vi "Mavlink Message Read.vi"(8 "error_in":errorcluster, 11 "VISA in":refnum<visa-resource-name>) -> (0 "error_out":errorcluster, 2 "mav_msg":T2, 3 "VISA out":refnum<visa-resource-name>)   [LabVIEW 2023]
panel:
  out "crc_counter":u32
  out "packet_counter":u32
  out "mav_msg_array":T1(array[cluster])
  out "check_mav_msg_array":bool
  out "CRC":bool
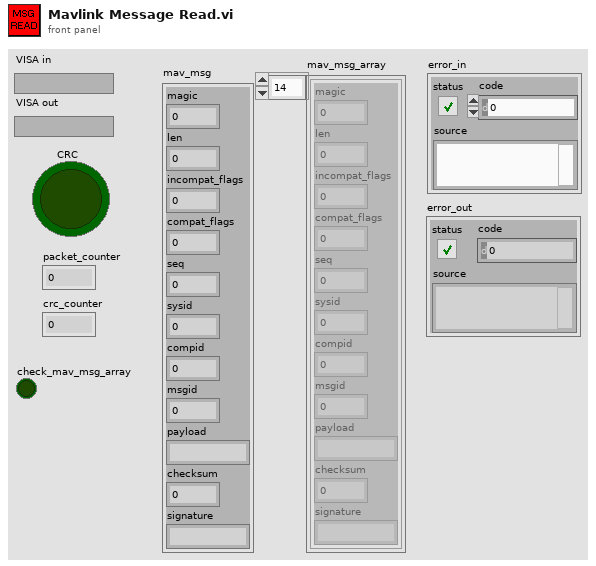
[diagram p1: front panel]
types:
  T1 = cluster{"len":u8, "incompat_flags":u8, "compat_flags":u8, "seq":u8, "sysid":u8, "compid":u8, "msgid":u32, "magic":u8, "payload":string, "checksum":u16, "signature":string}[]
  T2 = cluster{"len":u8, "incompat_flags":u8, "compat_flags":u8, "seq":u8, "sysid":u8, "compid":u8, "msgid":u32, "magic":u8, "payload":string, "checksum":u16, "signature":string}
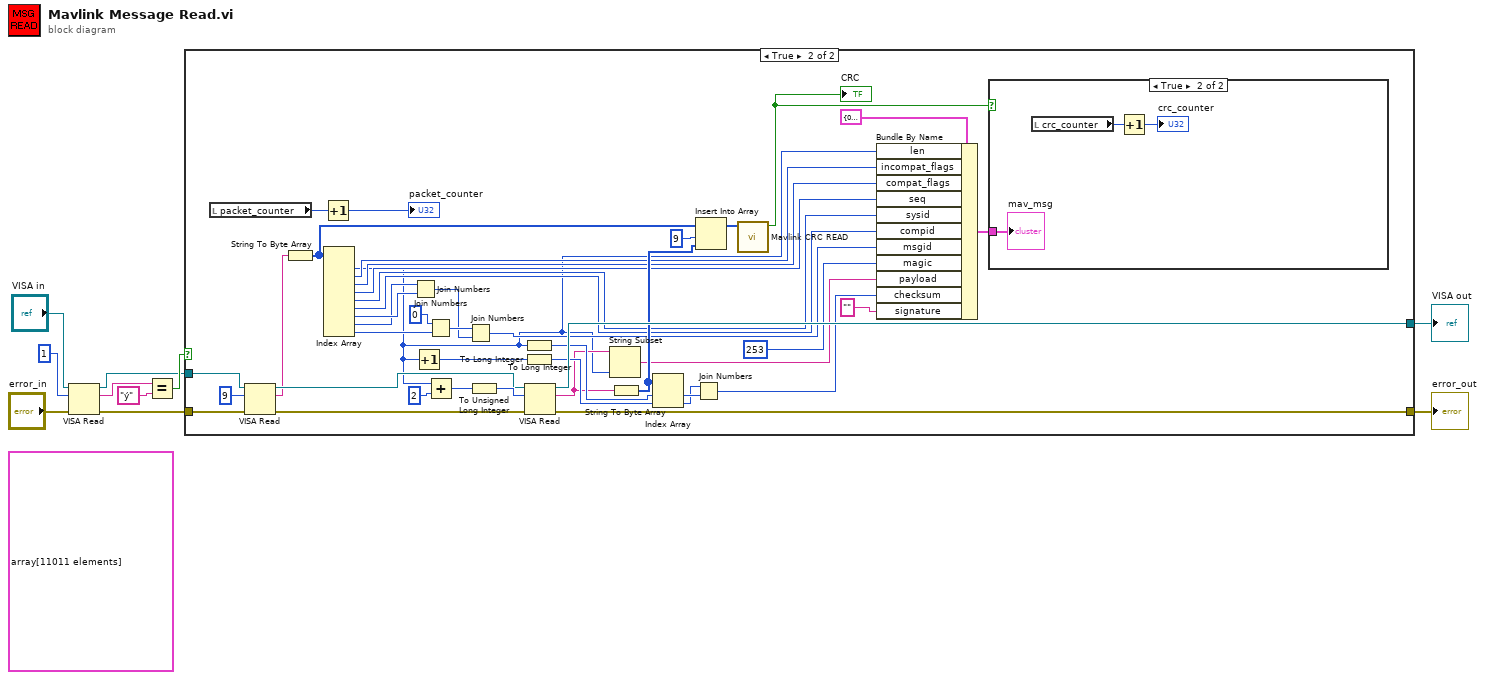
[diagram p0: block diagram]
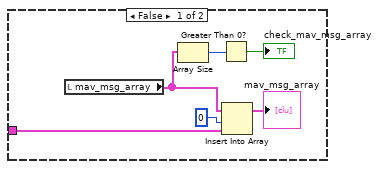
[diagram p3: hidden frame]
diagram:
  (unwired) T1 array[11011 elements] ("mav_msg_array")
  n1 = VISA Read(VISA resource name="VISA in", byte count=u32 1, error in (no error)="error_in") -> (VISA resource name out=w7:refnum<visa-resource-name>, read buffer=w9:string, error out=w8:errorcluster)  [unwired: 1 out]
  n2 = Equal?(x=w9, y="ý") -> (x = y?=w10:bool)
  n3 = case shown="True" w10 {
    tunnel: w7 -> [w11 w53]
    tunnel: w8 -> [w12 w54]
    tunnel: [w12 w27] -> w3
    tunnel: [w11 w55] -> w1
    frame False {
    }
    frame True {
      n4 = local read "packet_counter"() -> (w52:u32)
      n5 = VISA Read(VISA resource name=w53, byte count=u32 9, error in (no error)=w54) -> (VISA resource name out=w35:refnum<visa-resource-name>, read buffer=w34:string, error out=w36:errorcluster)  [unwired: 1 out]
      n6 = String To Byte Array(string=w34) -> (unsigned byte array=w37:u8[])
      n7 = Increment(x=w52) -> (x+1=→"packet_counter":u32)
      n8 = Index Array(array=w37) -> (element #1=w13:u8, element #2=w25:u8, element #3=w24:u8, element #4=w23:u8, element #5=w22:u8, element #6=w21:u8, element #7=w48:u8, element #8=w47:u8, element #9=w46:u8)  [unwired: 9 in]
      n9 = Join Numbers(hi=w47, lo=w48) -> ((hi.lo)=w43:u16)
      n10 = Increment(x=w13) -> (x+1=w39:u8)
      n11 = Join Numbers(hi=u8 0, lo=w46) -> ((hi.lo)=w44:u16)
      n12 = Add(x=w13, y=u8 2) -> (x+y=w41:u8)
      n13 = Join Numbers(hi=w44, lo=w43) -> ((hi.lo)=w20:u32)
      n14 = To Unsigned Long Integer(number=w41) -> (unsigned 32bit integer=w42:u32)
      n15 = To Long Integer(number=w13) -> (32bit integer=w38:i32)
      n16 = To Long Integer(number=w39) -> (32bit integer=w40:i32)
      n17 = VISA Read(VISA resource name=w35, byte count=w42, error in (no error)=w36) -> (VISA resource name out=w55:refnum<visa-resource-name>, read buffer=w29:string, error out=w27:errorcluster)  [unwired: 1 out]
      n18 = String Subset(string=w29, length (rest)=w13) -> (substring=w19:string)  [unwired: 1 in]
      n19 = String To Byte Array(string=w29) -> (unsigned byte array=w33:u8[])
      n20 = Index Array(array=w33, index #1=w38, index #2=w40) -> (element #1=w31:u8, element #2=w30:u8)
      n21 = Join Numbers(hi=w30, lo=w31) -> ((hi.lo)=w18:u16)
      n22 = Insert Into Array(array=w37, index=9, new element=w33) -> (w51:u8[])
      n23 = call "Mavlink CRC READ.vi"("Byte IN"=w51) -> ("CRC"=w28:bool)  [unwired: 10 in]
      "CRC" <- w28
      n24 = Bundle By Name(cluster=T2 {"len"=0, "incompat_flags"=0, "compat_flags"=0, "seq"=0, "sysid"=0, "compid"=0, "msgid"=0, "magic"=0, "payload"="", "checksum"=0, "signature"=""} ("mav_msg"), "len"=w13, "incompat_flags"=w25, "compat_flags"=w24, "seq"=w23, "sysid"=w22, "compid"=w21, "msgid"=w20, "magic"=u8 253, "payload"=w19, "checksum"=w18, "signature"="") -> (w14:T2)
      n25 = case shown="True" w28 {
        tunnel: w14 -> [w60 w64]
        frame False {
          n26 = local read "mav_msg_array"() -> (w58:T1)
          n27 = Array Size(array=w58) -> (size(s)=w59:i32)
          n28 = Greater Than 0?(x=w59) -> (x > 0?=→"check_mav_msg_array":bool)
          n29 = Insert Into Array(array=w58, index=0, new element=w60) -> (→"mav_msg_array":T1)
        }
        frame True {
          n30 = local read "crc_counter"() -> (w63:u32)
          n31 = Increment(x=w63) -> (x+1=→"crc_counter":u32)
          "mav_msg" <- w64
        }
      }
    }
  }
  "error_out" <- w3
  "VISA out" <- w1
